vi "Disconnect.vi"(8 "error in (no error)":errorcluster, 11 "UDP in":refnum<class "UDP.lvclass">) -> (0 "error out":errorcluster, 3 "UDP out":refnum<class "UDP.lvclass">)   [LabVIEW 2018, in "UDP.lvlib" / "UDP.lvclass"]
uses:
  UDP.lvclass
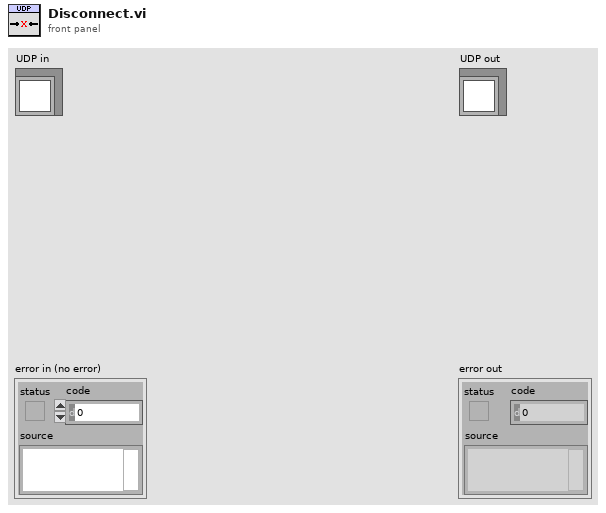
[diagram p1: front panel]
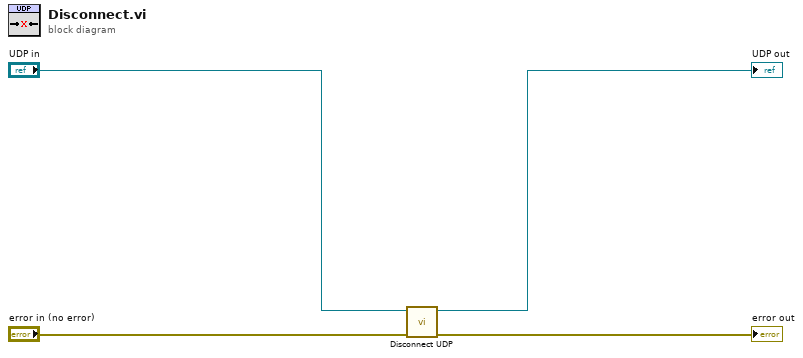
[diagram p0: block diagram]
diagram:
  n1 = call-dynamic "Disconnect UDP.vi"("error in (no error)"="error in (no error)", "UDP in"="UDP in") -> ("error out"=→"error out":errorcluster, "UDP out"=→"UDP out":refnum<class "UDP.lvclass">)  [unwired: 8 in]
